vi "GeoData.vi"() -> ()   [LabVIEW 2017] (continued)
NY\tSuffolk County\tH1\n11752\t36103\tIslip terrace\tNY\tSuffolk County\tH1\n11767\t36103\tNesconset\tNY\tSuffolk County\tH1\n11780\t36103\tSaint james\tNY\tSuffolk County\tH1\n11776\t36103\tPort jefferson station\tNY\tSuffolk County\tH1\n11786\t36103\tShoreham\tNY\tSuffolk County\tH1\n11901\t36103\tRiverhead\tNY\tSuffolk County\tH1\n11942\t36103\tEast quogue\tNY\tSuffolk County\tH1\n11963\t36103\tSag harbor\tNY\tSuffolk County\tH1\n11940\t36103\tEast moriches\tNY\tSuffolk County\tH1\n11941\t36103\tEastport\tNY\tSuffolk County\tH1\n11962\t36103\tSagaponack\tNY\tSuffolk County\tH1\n11770\t36103\tOcean beach\tNY\tSuffolk County\tH1\n11965\t36103\tShelter island heights\tNY\tSuffolk County\tH1\n11947\t36103\tJamesport\tNY\tSuffolk County\tH1\n11706\t36103\tBay shore\tNY\tSuffolk County\tH1\n11720\t36103\tCentereach\tNY\tSuffolk County\tH1\n11718\t36103\tBrightwaters\tNY\tSuffolk County\tH1\n11763\t36103\tMedford\tNY\tSuffolk County\tH1\n11768\t36103\tNorthport\tNY\tSuffolk County\tH1\n11766\t36103\tMount sinai\tNY\tSuffolk County\tH1\n11779\t36103\tRonkonkoma\tNY\tSuffolk County\tH1\n11787\t36103\tSmithtown\tNY\tSuffolk County\tH1\n11937\t36103\tEast hampton\tNY\tSuffolk County\tH1\n11944\t36103\tGreenport\tNY\tSuffolk County\tH1\n11957\t36103\tOrient\tNY\tSuffolk County\tH1\n11954\t36103\tMontauk\tNY\tSuffolk County\tH1\n11960\t36103\tRemsenburg\tNY\tSuffolk County\tH1\n11969\t36103\tSouthampton\tNY\tSuffolk County\tH1\n11939\t36103\tEast marion\tNY\tSuffolk County\tH1\n11964\t36103\tShelter island\tNY\tSuffolk County\tH1\n12566\t36105\tPine bush\tNY\tSullivan County\tH1\n12742\t36105\tHarris\tNY\tSullivan County\tH1\n12732\t36105\tEldred\tNY\tSullivan County\tH1\n12745\t36105\tHortonville\tNY\tSullivan County\tH1\n12720\t36105\tBethel\tNY\tSullivan County\tH1\n12758\t36105\tLivingston manor\tNY\tSullivan County\tH1\n12458\t36105\tNapanoch\tNY\tSullivan County\tH1\n12762\t36105\tMongaup valley\tNY\tSullivan County\tH1\n12777\t36105\tForestburgh\tNY\tSullivan County\tH1\n12775\t36105\tRock hill\tNY\tSullivan County\tH1\n12763\t36105\tMountain dale\tNY\tSullivan County\tH1\n12743\t36105\tHighland lake\tNY\tSullivan County\tH1\n12767\t36105\tObernburg\tNY\tSullivan County\tH1\n12729\t36105\tCuddebackville\tNY\tSullivan County\tH1\n12748\t36105\tJeffersonville\tNY\tSullivan County\tH1\n12723\t36105\tCallicoon\tNY\tSullivan County\tH1\n12776\t36105\tRoscoe\tNY\tSullivan County\tH1\n12766\t36105\tNorth branch\tNY\tSullivan County\tH1\n12736\t36105\tFremont center\tNY\tSullivan County\tH1\n12722\t36105\tBurlingham\tNY\tSullivan County\tH1\n12721\t36105\tBloomingburg\tNY\tSullivan County\tH1\n12725\t36105\tClaryville\tNY\tSullivan County\tH1\n12726\t36105\tCochecton\tNY\tSullivan County\tH1\n12791\t36105\tYoungsville\tNY\tSullivan County\tH1\n12733\t36105\tFallsburg\tNY\tSullivan County\tH1\n12750\t36105\tKenoza lake\tNY\tSullivan County\tH1\n12724\t36105\tCallicoon center\tNY\tSullivan County\tH1\n12781\t36105\tSummitville\tNY\tSullivan County\tH1\n10940\t36105\tMiddletown\tNY\tSullivan County\tH1\n12701\t36105\tMonticello\tNY\tSullivan County\tH1\n12754\t36105\tLiberty\tNY\tSullivan County\tH1\n12741\t36105\tHankins\tNY\tSullivan County\tH1\n12738\t36105\tGlen wild\tNY\tSullivan County\tH1\n12783\t36105\tSwan lake\tNY\tSullivan County\tH1\n12740\t36105\tGrahamsville\tNY\tSullivan County\tH1\n12759\t36105\tLoch sheldrake\tNY\tSullivan County\tH1\n12786\t36105\tWhite lake\tNY\tSullivan County\tH1\n12787\t36105\tWhite sulphur springs\tNY\tSullivan County\tH1\n12435\t36105\tGreenfield park\tNY\tSullivan County\tH1\n12737\t36105\tGlen spey\tNY\tSullivan County\tH1\n12790\t36105\tWurtsboro\tNY\tSullivan County\tH1\n12768\t36105\tParksville\tNY\tSullivan County\tH1\n12779\t36105\tSouth fallsburg\tNY\tSullivan County\tH1\n12789\t36105\tWoodridge\tNY\tSullivan County\tH1\n12751\t36105\tKiamesha lake\tNY\tSullivan County\tH1\n12752\t36105\tLake huntington\tNY\tSullivan County\tH1\n12749\t36105\tKauneonga lake\tNY\tSullivan County\tH1\n12769\t36105\tPhillipsport\tNY\tSullivan County\tH1\n12784\t36105\tThompsonville\tNY\tSullivan County\tH1\n10963\t36105\tOtisville\tNY\tSullivan County\tH1\n12764\t36105\tNarrowsburg\tNY\tSullivan County\tH1\n12760\t36105\tLong eddy\tNY\tSullivan County\tH1\n12780\t36105\tSparrow bush\tNY\tSullivan County\tH1\n12788\t36105\tWoodbourne\tNY\tSullivan County\tH1\n12734\t36105\tFerndale\tNY\tSullivan County\tH1\n12765\t36105\tNeversink\tNY\tSullivan County\tH1\n12770\t36105\tPond eddy\tNY\tSullivan County\tH1\n12747\t36105\tHurleyville\tNY\tSullivan County\tH1\n12719\t36105\tBarryville\tNY\tSullivan County\tH1\n12792\t36105\tYulan\tNY\tSullivan County\tH1\n12778\t36105\tSmallwood\tNY\tSullivan County\tH1\n13850\t36107\tVestal\tNY\tTioga County\tH1\n13835\t36107\tRichford\tNY\tTioga County\tH1\n13864\t36107\tWillseyville\tNY\tTioga County\tH1\n13840\t36107\tSmithboro\tNY\tTioga County\tH1\n13845\t36107\tTioga center\tNY\tTioga County\tH1\n13732\t36107\tApalachin\tNY\tTioga County\tH1\n14889\t36107\tVan etten\tNY\tTioga County\tH1\n14883\t36107\tSpencer\tNY\tTioga County\tH1\n13734\t36107\tBarton\tNY\tTioga County\tH1\n13736\t36107\tBerkshire\tNY\tTioga County\tH1\n13811\t36107\tNewark valley\tNY\tTioga County\tH1\n13827\t36107\tOwego\tNY\tTioga County\tH1\n14859\t36107\tLockwood\tNY\tTioga County\tH1\n13743\t36107\tCandor\tNY\tTioga County\tH1\n13760\t36107\tEndicott\tNY\tTioga County\tH1\n14817\t36107\tBrooktondale\tNY\tTioga County\tH1\n14892\t36107\tWaverly\tNY\tTioga County\tH1\n13812\t36107\tNichols\tNY\tTioga County\tH1\n13053\t36109\tDryden\tNY\tTompkins County\tH1\n13092\t36109\tLocke\tNY\tTompkins County\tH1\n13864\t36109\tWillseyville\tNY\tTompkins County\tH1\n14867\t36109\tNewfield\tNY\tTompkins County\tH1\n14853\t36109\tIthaca\tNY\tTompkins County\tH1\n14883\t36109\tSpencer\tNY\tTompkins County\tH1\n13736\t36109\tBerkshire\tNY\tTompkins County\tH1\n14882\t36109\tLansing\tNY\tTompkins County\tH1\n13045\t36109\tCortland\tNY\tTompkins County\tH1\n13068\t36109\tFreeville\tNY\tTompkins County\tH1\n13073\t36109\tGroton\tNY\tTompkins County\tH1\n13062\t36109\tEtna\tNY\tTompkins County\tH1\n14854\t36109\tJacksonville\tNY\tTompkins County\tH1\n14817\t36109\tBrooktondale\tNY\tTompkins County\tH1\n14886\t36109\tTrumansburg\tNY\tTompkins County\tH1\n13081\t36109\tKing ferry\tNY\tTompkins County\tH1\n13102\t36109\tMc lean\tNY\tTompkins County\tH1\n14881\t36109\tSlaterville springs\tNY\tTompkins County\tH1\n14850\t36109\tIthaca\tNY\tTompkins County\tH1\n14851\t36109\tIthaca\tNY\tTompkins County\tH1\n14852\t36109\tIthaca\tNY\tTompkins County\tH1\n12455\t36111\tMargaretville\tNY\tUlster County\tH1\n12466\t36111\tPort ewen\tNY\tUlster County\tH1\n12443\t36111\tHurley\tNY\tUlster County\tH1\n12404\t36111\tAccord\tNY\tUlster County\tH1\n12494\t36111\tWest shokan\tNY\tUlster County\tH1\n12515\t36111\tClintondale\tNY\tUlster County\tH1\n12566\t36111\tPine bush\tNY\tUlster County\tH1\n13731\t36111\tAndes\tNY\tUlster County\tH1\n12409\t36111\tBearsville\tNY\tUlster County\tH1\n12589\t36111\tWallkill\tNY\tUlster County\tH1\n12406\t36111\tArkville\tNY\tUlster County\tH1\n12419\t36111\tCottekill\tNY\tUlster County\tH1\n12448\t36111\tLake hill\tNY\tUlster County\tH1\n12457\t36111\tMount tremper\tNY\tUlster County\tH1\n12588\t36111\tWalker valley\tNY\tUlster County\tH1\n12446\t36111\tKerhonkson\tNY\tUlster County\tH1\n12464\t36111\tPhoenicia\tNY\tUlster County\tH1\n12461\t36111\tOlivebridge\tNY\tUlster County\tH1\n12525\t36111\tGardiner\tNY\tUlster County\tH1\n12561\t36111\tNew paltz\tNY\tUlster County\tH1\n12586\t36111\tWalden\tNY\tUlster County\tH1\n12758\t36111\tLivingston manor\tNY\tUlster County\tH1\n12458\t36111\tNapanoch\tNY\tUlster County\tH1\n12471\t36111\tRifton\tNY\tUlster County\tH1\n12410\t36111\tBig indian\tNY\tUlster County\tH1\n12475\t36111\tRuby\tNY\tUlster County\tH1\n12417\t36111\tConnelly\tNY\tUlster County\tH1\n12428\t36111\tEllenville\tNY\tUlster County\tH1\n12472\t36111\tRosendale\tNY\tUlster County\tH1\n12481\t36111\tShokan\tNY\tUlster County\tH1\n12763\t36111\tMountain dale\tNY\tUlster County\tH1\n12441\t36111\tHighmount\tNY\tUlster County\tH1\n12548\t36111\tModena\tNY\tUlster County\tH1\n12490\t36111\tWest camp\tNY\tUlster County\tH1\n12486\t36111\tTillson\tNY\tUlster County\tH1\n12477\t36111\tSaugerties\tNY\tUlster County\tH1\n12414\t36111\tCatskill\tNY\tUlster County\tH1\n12402\t36111\tKingston\tNY\tUlster County\tH1\n12491\t36111\tWest hurley\tNY\tUlster County\tH1\n12542\t36111\tMarlboro\tNY\tUlster County\tH1\n12498\t36111\tWoodstock\tNY\tUlster County\tH1\n12487\t36111\tUlster park\tNY\tUlster County\tH1\n12725\t36111\tClaryville\tNY\tUlster County\tH1\n12433\t36111\tGlenford\tNY\tUlster County\tH1\n12480\t36111\tShandaken\tNY\tUlster County\tH1\n12456\t36111\tMount marion\tNY\tUlster County\tH1\n12429\t36111\tEsopus\tNY\tUlster County\tH1\n12401\t36111\tKingston\tNY\tUlster County\tH1\n12528\t36111\tHighland\tNY\tUlster County\tH1\n12465\t36111\tPine hill\tNY\tUlster County\tH1\n12740\t36111\tGrahamsville\tNY\tUlster County\tH1\n12453\t36111\tMalden on hudson\tNY\tUlster County\tH1\n12411\t36111\tBloomington\tNY\tUlster County\tH1\n12495\t36111\tWillow\tNY\tUlster County\tH1\n12435\t36111\tGreenfield park\tNY\tUlster County\tH1\n12432\t36111\tGlasco\tNY\tUlster County\tH1\n12483\t36111\tSpring glen\tNY\tUlster County\tH1\n12789\t36111\tWoodridge\tNY\tUlster County\tH1\n12489\t36111\tWawarsing\tNY\tUlster County\tH1\n12416\t36111\tChichester\tNY\tUlster County\tH1\n12568\t36111\tPlattekill\tNY\tUlster County\tH1\n12493\t36111\tWest park\tNY\tUlster County\tH1\n12420\t36111\tCragsmoor\tNY\tUlster County\tH1\n12463\t36111\tPalenville\tNY\tUlster County\tH1\n12440\t36111\tHigh falls\tNY\tUlster County\tH1\n12449\t36111\tLake katrine\tNY\tUlster County\tH1\n12484\t36111\tStone ridge\tNY\tUlster County\tH1\n12547\t36111\tMilton\tNY\tUlster County\tH1\n12412\t36111\tBoiceville\tNY\tUlster County\tH1\n12856\t36113\tNorth river\tNY\tWarren County\tH1\n12844\t36113\tKattskill bay\tNY\tWarren County\tH1\n12814\t36113\tBolton landing\tNY\tWarren County\tH1\n12885\t36113\tWarrensburg\tNY\tWarren County\tH1\n12817\t36113\tChestertown\tNY\tWarren County\tH1\n12878\t36113\tStony creek\tNY\tWarren County\tH1\n12810\t36113\tAthol\tNY\tWarren County\tH1\n12808\t36113\tAdirondack\tNY\tWarren County\tH1\n12835\t36113\tHadley\tNY\tWarren County\tH1\n12857\t36113\tOlmstedville\tNY\tWarren County\tH1\n12862\t36113\tRiparius\tNY\tWarren County\tH1\n12839\t36113\tHudson falls\tNY\tWarren County\tH1\n12824\t36113\tDiamond point\tNY\tWarren County\tH1\n12804\t36113\tQueensbury\tNY\tWarren County\tH1\n12815\t36113\tBrant lake\tNY\tWarren County\tH1\n12836\t36113\tHague\tNY\tWarren County\tH1\n12820\t36113\tCleverdale\tNY\tWarren County\tH1\n12870\t36113\tSchroon lake\tNY\tWarren County\tH1\n12886\t36113\tWevertown\tNY\tWarren County\tH1\n12845\t36113\tLake george\tNY\tWarren County\tH1\n12853\t36113\tNorth creek\tNY\tWarren County\tH1\n12843\t36113\tJohnsburg\tNY\tWarren County\tH1\n12860\t36113\tPottersville\tNY\tWarren County\tH1\n12874\t36113\tSilver bay\tNY\tWarren County\tH1\n12803\t36113\tSouth glens falls\tNY\tWarren County\tH1\n12801\t36113\tGlens falls\tNY\tWarren County\tH1\n12846\t36113\tLake luzerne\tNY\tWarren County\tH1\n12811\t36113\tBakers mills\tNY\tWarren County\tH1\n12828\t36115\tFort edward\tNY\tWashington County\tH1\n12883\t36115\tTiconderoga\tNY\tWashington County\tH1\n12841\t36115\tHuletts landing\tNY\tWashington County\tH1\n12844\t36115\tKattskill bay\tNY\tWashington County\tH1\n12185\t36115\tValley falls\tNY\tWashington County\tH1\n12849\t36115\tMiddle granville\tNY\tWashington County\tH1\n12028\t36115\tBuskirk\tNY\tWashington County\tH1\n12094\t36115\tJohnsonville\tNY\tWashington County\tH1\n12834\t36115\tGreenwich\tNY\tWashington County\tH1\n12838\t36115\tHartford\tNY\tWashington County\tH1\n12887\t36115\tWhitehall\tNY\tWashington County\tH1\n12837\t36115\tHampton\tNY\tWashington County\tH1\n12861\t36115\tPutnam station\tNY\tWashington County\tH1\n12823\t36115\tCossayuna\tNY\tWashington County\tH1\n12848\t36115\tMiddle falls\tNY\tWashington County\tH1\n12057\t36115\tEagle bridge\tNY\tWashington County\tH1\n12839\t36115\tHudson falls\tNY\tWashington County\tH1\n12804\t36115\tQueensbury\tNY\tWashington County\tH1\n12865\t36115\tSalem\tNY\tWashington County\tH1\n12873\t36115\tShushan\tNY\tWashington County\tH1\n12090\t36115\tHoosick falls\tNY\tWashington County\tH1\n12816\t36115\tCambridge\tNY\tWashington County\tH1\n12809\t36115\tArgyle\tNY\tWashington County\tH1\n12832\t36115\tGranville\tNY\tWashington County\tH1\n12821\t36115\tComstock\tNY\tWashington County\tH1\n12854\t36115\tNorth granville\tNY\tWashington County\tH1\n12827\t36115\tFort ann\tNY\tWashington County\tH1\n12154\t36115\tSchaghticoke\tNY\tWashington County\tH1\n12819\t36115\tClemons\tNY\tWashington County\tH1\n13143\t36117\tRed creek\tNY\tWayne County\tH1\n14433\t36117\tClyde\tNY\tWayne County\tH1\n14580\t36117\tWebster\tNY\tWayne County\tH1\n14563\t36117\tUnion hill\tNY\tWayne County\tH1\n14502\t36117\tMacedon\tNY\tWayne County\tH1\n14555\t36117\tSodus point\tNY\tWayne County\tH1\n14542\t36117\tRose\tNY\tWayne County\tH1\n14519\t36117\tOntario\tNY\tWayne County\tH1\n14413\t36117\tAlton\tNY\tWayne County\tH1\n13148\t36117\tSeneca falls\tNY\tWayne County\tH1\n14450\t36117\tFairport\tNY\tWayne County\tH1\n14589\t36117\tWilliamson\tNY\tWayne County\tH1\n13146\t36117\tSavannah\tNY\tWayne County\tH1\n14505\t36117\tMarion\tNY\tWayne County\tH1\n14513\t36117\tNewark\tNY\tWayne County\tH1\n13154\t36117\tSouth butler\tNY\tWayne County\tH1\n13156\t36117\tSterling\tNY\tWayne County\tH1\n14432\t36117\tClifton springs\tNY\tWayne County\tH1\n14489\t36117\tLyons\tNY\tWayne County\tH1\n14516\t36117\tNorth rose\tNY\tWayne County\tH1\n14522\t36117\tPalmyra\tNY\tWayne County\tH1\n14551\t36117\tSodus\tNY\tWayne County\tH1\n14538\t36117\tPultneyville\tNY\tWayne County\tH1\n13165\t36117\tWaterloo\tNY\tWayne County\tH1\n14532\t36117\tPhelps\tNY\tWayne County\tH1\n14590\t36117\tWolcott\tNY\tWayne County\tH1\n14568\t36117\tWalworth\tNY\tWayne County\tH1\n14520\t36117\tOntario center\tNY\tWayne County\tH1\n14449\t36117\tEast williamson\tNY\tWayne County\tH1\n10511\t36119\tBuchanan\tNY\tWestchester County\tH1\n10547\t36119\tMohegan lake\tNY\tWestchester County\tH1\n10580\t36119\tRye\tNY\tWestchester County\tH1\n10594\t36119\tThornwood\tNY\tWestchester County\tH1\n10601\t36119\tWhite plains\tNY\tWestchester County\tH1\n10704\t36119\tYonkers\tNY\tWestchester County\tH1\n10801\t36119\tNew rochelle\tNY\tWestchester County\tH1\n10466\t36119\tBronx\tNY\tWestchester County\tH1\n10510\t36119\tBriarcliff manor\tNY\tWestchester County\tH1\n10504\t36119\tArmonk\tNY\tWestchester County\tH1\n10550\t36119\tMount vernon\tNY\tWestchester County\tH1\n10528\t36119\tHarrison\tNY\tWestchester County\tH1\n10589\t36119\tSomers\tNY\tWestchester County\tH1\n10802\t36119\tNew rochelle\tNY\tWestchester County\tH1\n10535\t36119\tJefferson valley\tNY\tWestchester County\tH1\n10545\t36119\tMaryknoll\tNY\tWestchester County\tH1\n10507\t36119\tBedford hills\tNY\tWestchester County\tH1\n10509\t36119\tBrewster\tNY\tWestchester County\tH1\n10573\t36119\tPort chester\tNY\tWestchester County\tH1\n10605\t36119\tWhite plains\tNY\tWestchester County\tH1\n10706\t36119\tHastings on hudson\tNY\tWestchester County\tH1\n10710\t36119\tYonkers\tNY\tWestchester County\tH1\n10505\t36119\tBaldwin place\tNY\tWestchester County\tH1\n10520\t36119\tCroton on hudson\tNY\tWestchester County\tH1\n10514\t36119\tChappaqua\tNY\tWestchester County\tH1\n10502\t36119\tArdsley\tNY\tWestchester County\tH1\n10538\t36119\tLarchmont\tNY\tWestchester County\tH1\n10549\t36119\tMount kisco\tNY\tWestchester County\tH1\n10523\t36119\tElmsford\tNY\tWestchester County\tH1\n10536\t36119\tKatonah\tNY\tWestchester County\tH1\n10533\t36119\tIrvington\tNY\tWestchester County\tH1\n10570\t36119\tPleasantville\tNY\tWestchester County\tH1\n10578\t36119\tPurdys\tNY\tWestchester County\tH1\n10709\t36119\tEastchester\tNY\tWestchester County\tH1\n10560\t36119\tNorth salem\tNY\tWestchester County\tH1\n10526\t36119\tGoldens bridge\tNY\tWestchester County\tH1\n10587\t36119\tShenorock\tNY\tWestchester County\tH1\n10506\t36119\tBedford\tNY\tWestchester County\tH1\n10532\t36119\tHawthorne\tNY\tWestchester County\tH1\n10603\t36119\tWhite plains\tNY\tWestchester County\tH1\n10591\t36119\tTarrytown\tNY\tWestchester County\tH1\n10701\t36119\tYonkers\tNY\tWestchester County\tH1\n10607\t36119\tWhite plains\tNY\tWestchester County\tH1\n10597\t36119\tWaccabuc\tNY\tWestchester County\tH1\n10610\t36119\tWhite plains\tNY\tWestchester County\tH1\n10503\t36119\tArdsley on hudson\tNY\tWestchester County\tH1\n10470\t36119\tBronx\tNY\tWestchester County\tH1\n10475\t36119\tBronx\tNY\tWestchester County\tH1\n10543\t36119\tMamaroneck\tNY\tWestchester County\tH1\n10541\t36119\tMahopac\tNY\tWestchester County\tH1\n10527\t36119\tGranite springs\tNY\tWestchester County\tH1\n10583\t36119\tScarsdale\tNY\tWestchester County\tH1\n10553\t36119\tMount vernon\tNY\tWestchester County\tH1\n10805\t36119\tNew rochelle\tNY\tWestchester County\tH1\n10708\t36119\tBronxville\tNY\tWestchester County\tH1\n10707\t36119\tTuckahoe\tNY\tWestchester County\tH1\n10577\t36119\tPurchase\tNY\tWestchester County\tH1\n10548\t36119\tMontrose\tNY\tWestchester County\tH1\n10562\t36119\tOssining\tNY\tWestchester County\tH1\n10566\t36119\tPeekskill\tNY\tWestchester County\tH1\n10552\t36119\tMount vernon\tNY\tWestchester County\tH1\n10606\t36119\tWhite plains\tNY\tWestchester County\tH1\n10705\t36119\tYonkers\tNY\tWestchester County\tH1\n10703\t36119\tYonkers\tNY\tWestchester County\tH1\n10588\t36119\tShrub oak\tNY\tWestchester County\tH1\n10501\t36119\tAmawalk\tNY\tWestchester County\tH1\n10540\t36119\tLincolndale\tNY\tWestchester County\tH1\n10518\t36119\tCross river\tNY\tWestchester County\tH1\n10519\t36119\tCroton falls\tNY\tWestchester County\tH1\n10522\t36119\tDobbs ferry\tNY\tWestchester County\tH1\n10530\t36119\tHartsdale\tNY\tWestchester County\tH1\n10546\t36119\tMillwood\tNY\tWestchester County\tH1\n10567\t36119\tCortlandt manor\tNY\tWestchester County\tH1\n10576\t36119\tPound ridge\tNY\tWestchester County\tH1\n10595\t36119\tValhalla\tNY\tWestchester County\tH1\n10598\t36119\tYorktown heights\tNY\tWestchester County\tH1\n10590\t36119\tSouth salem\tNY\tWestchester County\tH1\n10604\t36119\tWest harrison\tNY\tWestchester County\tH1\n10803\t36119\tPelham\tNY\tWestchester County\tH1\n10702\t36119\tYonkers\tNY\tWestchester County\tH1\n10804\t36119\tNew rochelle\tNY\tWestchester County\tH1\n10537\t36119\tLake peekskill\tNY\tWestchester County\tH1\n10551\t36119\tMount vernon\tNY\tWestchester County\tH1\n10517\t36119\tCrompond\tNY\tWestchester County\tH1\n10602\t36119\tWhite plains\tNY\tWestchester County\tH1\n10596\t36119\tVerplanck\tNY\tWestchester County\tH1\n14052\t36121\tEast aurora\tNY\tWyoming County\tH1\n14525\t36121\tPavilion\tNY\tWyoming County\tH1\n14037\t36121\tCowlesville\tNY\tWyoming County\tH1\n14549\t36121\tSilver lake\tNY\tWyoming County\tH1\n14030\t36121\tChaffee\tNY\tWyoming County\tH1\n14083\t36121\tJava village\tNY\tWyoming County\tH1\n14569\t36121\tWarsaw\tNY\tWyoming County\tH1\n14039\t36121\tDale\tNY\tWyoming County\tH1\n14113\t36121\tNorth java\tNY\tWyoming County\tH1\n14082\t36121\tJava center\tNY\tWyoming County\tH1\n14004\t36121\tAlden\tNY\tWyoming County\tH1\n14066\t36121\tGainesville\tNY\tWyoming County\tH1\n14427\t36121\tCastile\tNY\tWyoming County\tH1\n14591\t36121\tWyoming\tNY\tWyoming County\tH1\n14040\t36121\tDarien center\tNY\tWyoming County\tH1\n14145\t36121\tStrykersville\tNY\tWyoming County\tH1\n14533\t36121\tPiffard\tNY\tWyoming County\tH1\n14024\t36121\tBliss\tNY\tWyoming County\tH1\n14054\t36121\tEast bethany\tNY\tWyoming County\tH1\n14481\t36121\tLeicester\tNY\tWyoming County\tH1\n14009\t36121\tArcade\tNY\tWyoming County\tH1\n14011\t36121\tAttica\tNY\tWyoming County\tH1\n14550\t36121\tSilver springs\tNY\tWyoming County\tH1\n14735\t36121\tFillmore\tNY\tWyoming County\tH1\n14130\t36121\tPike\tNY\tWyoming County\tH1\n14167\t36121\tVarysburg\tNY\tWyoming County\tH1\n14530\t36121\tPerry\tNY\tWyoming County\tH1\n14536\t36121\tPortageville\tNY\tWyoming County\tH1\n14857\t36123\tLakemont\tNY\tYates County\tH1\n14512\t36123\tNaples\tNY\tYates County\tH1\n14837\t36123\tDundee\tNY\tYates County\tH1\n14544\t36123\tRushville\tNY\tYates County\tH1\n14478\t36123\tKeuka park\tNY\tYates County\tH1\n14441\t36123\tDresden\tNY\tYates County\tH1\n14424\t36123\tCanandaigua\tNY\tYates County\tH1\n14873\t36123\tPrattsburgh\tNY\tYates County\tH1\n14842\t36123\tHimrod\tNY\tYates County\tH1\n14418\t36123\tBranchport\tNY\tYates County\tH1\n14561\t36123\tStanley\tNY\tYates County\tH1\n14507\t36123\tMiddlesex\tNY\tYates County\tH1\n14878\t36123\tRock stream\tNY\tYates County\tH1\n14527\t36123\tPenn yan\tNY\tYates County\tH1\n14456\t36123\tGeneva\tNY\tYates County\tH1\n14415\t36123\tBellona\tNY\tYates County\tH1\n27201\t37001\tAlamance\tNC\tAlamance County\tH1\n27349\t37001\tSnow camp\tNC\tAlamance County\tH1\n27202\t37001\tAltamahaw\tNC\tAlamance County\tH1\n27344\t37001\tSiler city\tNC\tAlamance County\tH1\n27217\t37001\tBurlington\tNC\tAlamance County\tH1\n27258\t37001\tHaw river\tNC\tAlamance County\tH1\n27302\t37001\tMebane\tNC\tAlamance County\tH1\n27340\t37001\tSaxapahaw\tNC\tAlamance County\tH1\n27244\t37001\tElon\tNC\tAlamance County\tH1\n27253\t37001\tGraham\tNC\tAlamance County\tH1\n27216\t37001\tBurlington\tNC\tAlamance County\tH1\n27298\t37001\tLiberty\tNC\tAlamance County\tH1\n27359\t37001\tSwepsonville\tNC\tAlamance County\tH1\n27215\t37001\tBurlington\tNC\tAlamance County\tH1\n27249\t37001\tGibsonville\tNC\tAlamance County\tH1\n28636\t37003\tHiddenite\tNC\tAlexander County\tH1\n28681\t37003\tTaylorsville\tNC\tAlexander County\tH1\n28630\t37003\tGranite falls\tNC\tAlexander County\tH1\n28654\t37003\tMoravian falls\tNC\tAlexander County\tH1\n28601\t37003\tHickory\tNC\tAlexander County\tH1\n28625\t37003\tStatesville\tNC\tAlexander County\tH1\n28678\t37003\tStony point\tNC\tAlexander County\tH1\n28689\t37003\tUnion grove\tNC\tAlexander County\tH1\n28644\t37005\tLaurel springs\tNC\tAlleghany County\tH1\n28663\t37005\tPiney creek\tNC\tAlleghany County\tH1\n28675\t37005\tSparta\tNC\tAlleghany County\tH1\n28668\t37005\tRoaring gap\tNC\tAlleghany County\tH1\n28627\t37005\tGlade valley\tNC\tAlleghany County\tH1\n28672\t37005\tScottville\tNC\tAlleghany County\tH1\n27017\t37005\tDobson\tNC\tAlleghany County\tH1\n28631\t37005\tGrassy creek\tNC\tAlleghany County\tH1\n28623\t37005\tEnnice\tNC\tAlleghany County\tH1\n28007\t37007\tAnsonville\tNC\tAnson County\tH1\n28135\t37007\tPolkton\tNC\tAnson County\tH1\n28119\t37007\tMorven\tNC\tAnson County\tH1\n28091\t37007\tLilesville\tNC\tAnson County\tH1\n28133\t37007\tPeachland\tNC\tAnson County\tH1\n28102\t37007\tMc farlan\tNC\tAnson County\tH1\n28103\t37007\tMarshville\tNC\tAnson County\tH1\n28170\t37007\tWadesboro\tNC\tAnson County\tH1\n28644\t37009\tLaurel springs\tNC\tAshe County\tH1\n28640\t37009\tJefferson\tNC\tAshe County\tH1\n28698\t37009\tZionville\tNC\tAshe County\tH1\n28629\t37009\tGlendale springs\tNC\tAshe County\tH1\n28643\t37009\tLansing\tNC\tAshe County\tH1\n28626\t37009\tFleetwood\tNC\tAshe County\tH1\n28618\t37009\tDeep gap\tNC\tAshe County\tH1\n28684\t37009\tTodd\tNC\tAshe County\tH1\n28693\t37009\tWarrensville\tNC\tAshe County\tH1\n28672\t37009\tScottville\tNC\tAshe County\tH1\n28694\t37009\tWest jefferson\tNC\tAshe County\tH1\n28617\t37009\tCrumpler\tNC\tAshe County\tH1\n28631\t37009\tGrassy creek\tNC\tAshe County\tH1\n28615\t37009\tCreston\tNC\tAshe County\tH1\n28622\t37011\tElk park\tNC\tAvery County\tH1\n28664\t37011\tPlumtree\tNC\tAvery County\tH1\n28653\t37011\tMontezuma\tNC\tAvery County\tH1\n28604\t37011\tBanner elk\tNC\tAvery County\tH1\n28777\t37011\tSpruce pine\tNC\tAvery County\tH1\n28646\t37011\tLinville\tNC\tAvery County\tH1\n28607\t37011\tBoone\tNC\tAvery County\tH1\n28605\t37011\tBlowing rock\tNC\tAvery County\tH1\n28662\t37011\tPineola\tNC\tAvery County\tH1\n28611\t37011\tCollettsville\tNC\tAvery County\tH1\n28652\t37011\tMinneapolis\tNC\tAvery County\tH1\n28616\t37011\tCrossnore\tNC\tAvery County\tH1\n28657\t37011\tNewland\tNC\tAvery County\tH1\n28679\t37011\tSugar grove\tNC\tAvery County\tH1\n28705\t37011\tBakersville\tNC\tAvery County\tH1\n27806\t37013\tAurora\tNC\tBeaufort County\tH1\n27860\t37013\tPantego\tNC\tBeaufort County\tH1\n27814\t37013\tBlounts creek\tNC\tBeaufort County\tH1\n27810\t37013\tBelhaven\tNC\tBeaufort County\tH1\n27962\t37013\tPlymouth\tNC\tBeaufort County\tH1\n28586\t37013\tVanceboro\tNC\tBeaufort County\tH1\n27821\t37013\tEdward\tNC\tBeaufort County\tH1\n27837\t37013\tGrimesland\tNC\tBeaufort County\tH1\n27889\t37013\tWashington\tNC\tBeaufort County\tH1\n27808\t37013\tBath\tNC\tBeaufort County\tH1\n27817\t37013\tChocowinity\tNC\tBeaufort County\tH1\n27834\t37013\tGreenville\tNC\tBeaufort County\tH1\n27871\t37013\tRobersonville\tNC\tBeaufort County\tH1\n27865\t37013\tPinetown\tNC\tBeaufort County\tH1\n27957\t37015\tMerry hill\tNC\tBertie County\tH1\n27983\t37015\tWindsor\tNC\tBertie County\tH1\n27805\t37015\tAulander\tNC\tBertie County\tH1\n27967\t37015\tPowellsville\tNC\tBertie County\tH1\n27924\t37015\tColerain\tNC\tBertie County\tH1\n27872\t37015\tRoxobel\tNC\tBertie County\tH1\n27869\t37015\tRich square\tNC\tBertie County\tH1\n27910\t37015\tAhoskie\tNC\tBertie County\tH1\n27849\t37015\tLewiston woodville\tNC\tBertie County\tH1\n27847\t37015\tKelford\tNC\tBertie County\tH1\n28320\t37017\tBladenboro\tNC\tBladen County\tH1\n28448\t37017\tKelly\tNC\tBladen County\tH1\n28444\t37017\tHarrells\tNC\tBladen County\tH1\n28306\t37017\tFayetteville\tNC\tBladen County\tH1\n28456\t37017\tRiegelwood\tNC\tBladen County\tH1\n28392\t37017\tTar heel\tNC\tBladen County\tH1\n28435\t37017\tCurrie\tNC\tBladen County\tH1\n28384\t37017\tSaint pauls\tNC\tBladen County\tH1\n28423\t37017\tBolton\tNC\tBladen County\tH1\n28337\t37017\tElizabethtown\tNC\tBladen County\tH1\n28382\t37017\tRoseboro\tNC\tBladen County\tH1\n28434\t37017\tCouncil\tNC\tBladen County\tH1\n28447\t37017\tIvanhoe\tNC\tBladen County\tH1\n28332\t37017\tDublin\tNC\tBladen County\tH1\n28312\t37017\tFayetteville\tNC\tBladen County\tH1\n28399\t37017\tWhite oak\tNC\tBladen County\tH1\n28433\t37017\tClarkton\tNC\tBladen County\tH1\n28438\t37017\tEvergreen\tNC\tBladen County\tH1\n28441\t37017\tGarland\tNC\tBladen County\tH1\n28422\t37019\tBolivia\tNC\tBrunswick County\tH1\n28467\t37019\tCalabash\tNC\tBrunswick County\tH1\n28470\t37019\tShallotte\tNC\tBrunswick County\tH1\n28452\t37019\tLongwood\tNC\tBrunswick County\tH1\n28436\t37019\tDelco\tNC\tBrunswick County\tH1\n28456\t37019\tRiegelwood\tNC\tBrunswick County\tH1\n28479\t37019\tWinnabow\tNC\tBrunswick County\tH1\n28401\t37019\tWilmington\tNC\tBrunswick County\tH1\n28451\t37019\tLeland\tNC\tBrunswick County\tH1\n28462\t37019\tSupply\tNC\tBrunswick County\tH1\n28469\t37019\tOcean isle beach\tNC\tBrunswick County\tH1\n28459\t37019\tShallotte\tNC\tBrunswick County\tH1\n28420\t37019\tAsh\tNC\tBrunswick County\tH1\n28461\t37019\tSouthport\tNC\tBrunswick County\tH1\n28465\t37019\tOak island\tNC\tBrunswick County\tH1\n28468\t37019\tSunset beach\tNC\tBrunswick County\tH1\n28701\t37021\tAlexander\tNC\tBuncombe County\tH1\n28715\t37021\tCandler\tNC\tBuncombe County\tH1\n28730\t37021\tFairview\tNC\tBuncombe County\tH1\n28814\t37021\tAsheville\tNC\tBuncombe County\tH1\n28655\t37021\tMorganton\tNC\tBuncombe County\tH1\n28714\t37021\tBurnsville\tNC\tBuncombe County\tH1\n28721\t37021\tClyde\tNC\tBuncombe County\tH1\n28804\t37021\tAsheville\tNC\tBuncombe County\tH1\n28757\t37021\tMontreat\tNC\tBuncombe County\tH1\n28770\t37021\tRidgecrest\tNC\tBuncombe County\tH1\n28709\t37021\tBarnardsville\tNC\tBuncombe County\tH1\n28732\t37021\tFletcher\tNC\tBuncombe County\tH1\n28762\t37021\tOld fort\tNC\tBuncombe County\tH1\n28806\t37021\tAsheville\tNC\tBuncombe County\tH1\n28776\t37021\tSkyland\tNC\tBuncombe County\tH1\n28805\t37021\tAsheville\tNC\tBuncombe County\tH1\n28803\t37021\tAsheville\tNC\tBuncombe County\tH1\n28802\t37021\tAsheville\tNC\tBuncombe County\tH1\n28704\t37021\tArden\tNC\tBuncombe County\tH1\n28778\t37021\tSwannanoa\tNC\tBuncombe County\tH1\n28787\t37021\tWeaverville\tNC\tBuncombe County\tH1\n28711\t37021\tBlack mountain\tNC\tBuncombe County\tH1\n28716\t37021\tCanton\tNC\tBuncombe County\tH1\n28801\t37021\tAsheville\tNC\tBuncombe County\tH1\n28816\t37021\tAsheville\tNC\tBuncombe County\tH1\n28813\t37021\tAsheville\tNC\tBuncombe County\tH1\n28815\t37021\tAsheville\tNC\tBuncombe County\tH1\n28810\t37021\tAsheville\tNC\tBuncombe County\tH1\n28753\t37021\tMarshall\tNC\tBuncombe County\tH1\n28748\t37021\tLeicester\tNC\tBuncombe County\tH1\n28754\t37021\tMars hill\tNC\tBuncombe County\tH1\n28791\t37021\tHendersonville\tNC\tBuncombe County\tH1\n28728\t37021\tEnka\tNC\tBuncombe County\tH1\n28759\t37021\tMills river\tNC\tBuncombe County\tH1\n28792\t37021\tHendersonville\tNC\tBuncombe County\tH1\n28602\t37023\tHickory\tNC\tBurke County\tH1\n28666\t37023\tIcard\tNC\tBurke County\tH1\n28619\t37023\tDrexel\tNC\tBurke County\tH1\n28645\t37023\tLenoir\tNC\tBurke County\tH1\n28655\t37023\tMorganton\tNC\tBurke County\tH1\n28761\t37023\tNebo\tNC\tBurke County\tH1\n28641\t37023\tJonas ridge\tNC\tBurke County\tH1\n28647\t37023\tLinville falls\tNC\tBurke County\tH1\n28671\t37023\tRutherford college\tNC\tBurke County\tH1\n28628\t37023\tGlen alpine\tNC\tBurke County\tH1\n28612\t37023\tConnelly springs\tNC\tBurke County\tH1\n28680\t37023\tMorganton\tNC\tBurke County\tH1\n28018\t37023\tBostic\tNC\tBurke County\tH1\n28601\t37023\tHickory\tNC\tBurke County\tH1\n28637\t37023\tHildebran\tNC\tBurke County\tH1\n28690\t37023\tValdese\tNC\tBurke County\tH1\n28168\t37023\tVale\tNC\tBurke County\tH1\n28657\t37023\tNewland\tNC\tBurke County\tH1\n28090\t37023\tLawndale\tNC\tBurke County\tH1\n28026\t37025\tConcord\tNC\tCabarrus County\tH1\n28269\t37025\tCharlotte\tNC\tCabarrus County\tH1\n28027\t37025\tConcord\tNC\tCabarrus County\tH1\n28075\t37025\tHarrisburg\tNC\tCabarrus County\tH1\n28213\t37025\tCharlotte\tNC\tCabarrus County\tH1\n28227\t37025\tCharlotte\tNC\tCabarrus County\tH1\n28083\t37025\tKannapolis\tNC\tCabarrus County\tH1\n28097\t37025\tLocust\tNC\tCabarrus County\tH1\n28071\t37025\tGold hill\tNC\tCabarrus County\tH1\n28107\t37025\tMidland\tNC\tCabarrus County\tH1\n28138\t37025\tRockwell\tNC\tCabarrus County\tH1\n28124\t37025\tMount pleasant\tNC\tCabarrus County\tH1\n28025\t37025\tConcord\tNC\tCabarrus County\tH1\n28036\t37025\tDavidson\tNC\tCabarrus County\tH1\n28081\t37025\tKannapolis\tNC\tCabarrus County\tH1\n28215\t37025\tCharlotte\tNC\tCabarrus County\tH1\n28082\t37025\tKannapolis\tNC\tCabarrus County\tH1\n28078\t37025\tHuntersville\tNC\tCabarrus County\tH1\n28262\t37025\tCharlotte\tNC\tCabarrus County\tH1\n28624\t37027\tFerguson\tNC\tCaldwell County\tH1\n28645\t37027\tLenoir\tNC\tCaldwell County\tH1\n28655\t37027\tMorganton\tNC\tCaldwell County\tH1\n28681\t37027\tTaylorsville\tNC\tCaldwell County\tH1\n28633\t37027\tLenoir\tNC\tCaldwell County\tH1\n28661\t37027\tPatterson\tNC\tCaldwell County\tH1\n28638\t37027\tHudson\tNC\tCaldwell County\tH1\n28630\t37027\tGranite falls\tNC\tCaldwell County\tH1\n28605\t37027\tBlowing rock\tNC\tCaldwell County\tH1\n28601\t37027\tHickory\tNC\tCaldwell County\tH1\n28611\t37027\tCollettsville\tNC\tCaldwell County\tH1\n28606\t37027\tBoomer\tNC\tCaldwell County\tH1\n28667\t37027\tRhodhiss\tNC\tCaldwell County\tH1\n27973\t37029\tShawboro\tNC\tCamden County\tH1\n27921\t37029\tCamden\tNC\tCamden County\tH1\n27974\t37029\tShiloh\tNC\tCamden County\tH1\n27909\t37029\tElizabeth city\tNC\tCamden County\tH1\n27976\t37029\tSouth mills\tNC\tCamden County\tH1\n28511\t37031\tAtlantic\tNC\tCarteret County\tH1\n28528\t37031\tGloucester\tNC\tCarteret County\tH1\n28570\t37031\tNewport\tNC\tCarteret County\tH1\n28582\t37031\tStella\tNC\tCarteret County\tH1\n28531\t37031\tHarkers island\tNC\tCarteret County\tH1\n28584\t37031\tSwansboro\tNC\tCarteret County\tH1\n28553\t37031\tMarshallberg\tNC\tCarteret County\tH1\n28516\t37031\tBeaufort\tNC\tCarteret County\tH1\n28555\t37031\tMaysville\tNC\tCarteret County\tH1\n28524\t37031\tDavis\tNC\tCarteret County\tH1\n28579\t37031\tSmyrna\tNC\tCarteret County\tH1\n28520\t37031\tCedar island\tNC\tCarteret County\tH1\n28575\t37031\tSalter path\tNC\tCarteret County\tH1\n28512\t37031\tAtlantic beach\tNC\tCarteret County\tH1\n28577\t37031\tSealevel\tNC\tCarteret County\tH1\n28557\t37031\tMorehead city\tNC\tCarteret County\tH1\n28594\t37031\tEmerald isle\tNC\tCarteret County\tH1\n28581\t37031\tStacy\tNC\tCarteret County\tH1\n28532\t37031\tHavelock\tNC\tCarteret County\tH1\n27315\t37033\tProvidence\tNC\tCaswell County\tH1\n27343\t37033\tSemora\tNC\tCaswell County\tH1\n27212\t37033\tBlanch\tNC\tCaswell County\tH1\n27326\t37033\tRuffin\tNC\tCaswell County\tH1\n27320\t37033\tReidsville\tNC\tCaswell County\tH1\n27217\t37033\tBurlington\tNC\tCaswell County\tH1\n27379\t37033\tYanceyville\tNC\tCaswell County\tH1\n27302\t37033\tMebane\tNC\tCaswell County\tH1\n27244\t37033\tElon\tNC\tCaswell County\tH1\n27314\t37033\tProspect hill\tNC\tCaswell County\tH1\n27305\t37033\tMilton\tNC\tCaswell County\tH1\n27249\t37033\tGibsonville\tNC\tCaswell County\tH1\n27291\t37033\tLeasburg\tNC\tCaswell County\tH1\n27311\t37033\tPelham\tNC\tCaswell County\tH1\n28602\t37035\tHickory\tNC\tCatawba County\tH1\n28092\t37035\tLincolnton\tNC\tCatawba County\tH1\n28658\t37035\tNewton\tNC\tCatawba County\tH1\n28609\t37035\tCatawba\tNC\tCatawba County\tH1\n28650\t37035\tMaiden\tNC\tCatawba County\tH1\n28612\t37035\tConnelly springs\tNC\tCatawba County\tH1\n28673\t37035\tSherrills ford\tNC\tCatawba County\tH1\n28037\t37035\tDenver\tNC\tCatawba County\tH1\n28682\t37035\tTerrell\tNC\tCatawba County\tH1\n28603\t37035\tHickory\tNC\tCatawba County\tH1\n28601\t37035\tHickory\tNC\tCatawba County\tH1\n28610\t37035\tClaremont\tNC\tCatawba County\tH1\n28168\t37035\tVale\tNC\tCatawba County\tH1\n28613\t37035\tConover\tNC\tCatawba County\tH1\n28090\t37035\tLawndale\tNC\tCatawba County\tH1\n27349\t37037\tSnow camp\tNC\tChatham County\tH1\n27207\t37037\tBear creek\tNC\tChatham County\tH1\n27330\t37037\tSanford\tNC\tChatham County\tH1\n27344\t37037\tSiler city\tNC\tChatham County\tH1\n27502\t37037\tApex\tNC\tChatham County\tH1\n27519\t37037\tCary\tNC\tChatham County\tH1\n27562\t37037\tNew hill\tNC\tChatham County\tH1\n27325\t37037\tRobbins\tNC\tChatham County\tH1\n27713\t37037\tDurham\tNC\tChatham County\tH1\n27355\t37037\tStaley\tNC\tChatham County\tH1\n27252\t37037\tGoldston\tNC\tChatham County\tH1\n27312\t37037\tPittsboro\tNC\tChatham County\tH1\n27516\t37037\tChapel hill\tNC\tChatham County\tH1\n27256\t37037\tGulf\tNC\tChatham County\tH1\n27213\t37037\tBonlee\tNC\tChatham County\tH1\n27332\t37037\tSanford\tNC\tChatham County\tH1\n27523\t37037\tApex\tNC\tChatham County\tH1\n27517\t37037\tChapel hill\tNC\tChatham County\tH1\n27208\t37037\tBennett\tNC\tChatham County\tH1\n27298\t37037\tLiberty\tNC\tChatham County\tH1\n27540\t37037\tHolly springs\tNC\tChatham County\tH1\n27559\t37037\tMoncure\tNC\tChatham County\tH1\n28901\t37039\tAndrews\tNC\tCherokee County\tH1\n28905\t37039\tMarble\tNC\tCherokee County\tH1\n28903\t37039\tCulberson\tNC\tCherokee County\tH1\n28906\t37039\tMurphy\tNC\tCherokee County\tH1\n28902\t37039\tBrasstown\tNC\tCherokee County\tH1\n27946\t37041\tHobbsville\tNC\tChowan County\tH1\n27919\t37041\tBelvidere\tNC\tChowan County\tH1\n27980\t37041\tTyner\tNC\tChowan County\tH1\n27932\t37041\tEdenton\tNC\tChowan County\tH1\n28734\t37043\tFranklin\tNC\tClay County\tH1\n28906\t37043\tMurphy\tNC\tClay County\tH1\n28904\t37043\tHayesville\tNC\tClay County\tH1\n28902\t37043\tBrasstown\tNC\tClay County\tH1\n28909\t37043\tWarne\tNC\tClay County\tH1\n28073\t37045\tGrover\tNC\tCleveland County\tH1\n28042\t37045\tFallston\tNC\tCleveland County\tH1\n28612\t37045\tConnelly springs\tNC\tCleveland County\tH1\n28150\t37045\tShelby\tNC\tCleveland County\tH1\n28151\t37045\tShelby\tNC\tCleveland County\tH1\n28136\t37045\tPolkville\tNC\tCleveland County\tH1\n28021\t37045\tCherryville\tNC\tCleveland County\tH1\n28020\t37045\tCasar\tNC\tCleveland County\tH1\n28168\t37045\tVale\tNC\tCleveland County\tH1\n28017\t37045\tBoiling springs\tNC\tCleveland County\tH1\n28169\t37045\tWaco\tNC\tCleveland County\tH1\n28089\t37045\tLattimore\tNC\tCleveland County\tH1\n28152\t37045\tShelby\tNC\tCleveland County\tH1\n28040\t37045\tEllenboro\tNC\tCleveland County\tH1\n28086\t37045\tKings mountain\tNC\tCleveland County\tH1\n28090\t37045\tLawndale\tNC\tCleveland County\tH1\n28114\t37045\tMooresboro\tNC\tCleveland County\tH1\n28038\t37045\tEarl\tNC\tCleveland County\tH1\n28320\t37047\tBladenboro\tNC\tColumbus County\tH1\n28463\t37047\tTabor city\tNC\tColumbus County\tH1\n28436\t37047\tDelco\tNC\tColumbus County\tH1\n28455\t37047\tNakina\tNC\tColumbus County\tH1\n28456\t37047\tRiegelwood\tNC\tColumbus County\tH1\n28424\t37047\tBrunswick\tNC\tColumbus County\tH1\n28423\t37047\tBolton\tNC\tColumbus County\tH1\n28430\t37047\tCerro gordo\tNC\tColumbus County\tH1\n28431\t37047\tChadbourn\tNC\tColumbus County\tH1\n28472\t37047\tWhiteville\tNC\tColumbus County\tH1\n28433\t37047\tClarkton\tNC\tColumbus County\tH1\n28438\t37047\tEvergreen\tNC\tColumbus County\tH1\n28442\t37047\tHallsboro\tNC\tColumbus County\tH1\n28432\t37047\tClarendon\tNC\tColumbus County\tH1\n28450\t37047\tLake waccamaw\tNC\tColumbus County\tH1\n28439\t37047\tFair bluff\tNC\tColumbus County\tH1\n28530\t37049\tGrifton\tNC\tCraven County\tH1\n28501\t37049\tKinston\tNC\tCraven County\tH1\n28527\t37049\tErnul\tNC\tCraven County\tH1\n28560\t37049\tNew bern\tNC\tCraven County\tH1\n28573\t37049\tPollocksville\tNC\tCraven County\tH1\n28586\t37049\tVanceboro\tNC\tCraven County\tH1\n28533\t37049\tCherry point\tNC\tCraven County\tH1\n28526\t37049\tDover\tNC\tCraven County\tH1\n28561\t37049\tNew bern\tNC\tCraven County\tH1\n28563\t37049\tNew bern\tNC\tCraven County\tH1\n28564\t37049\tNew bern\tNC\tCraven County\tH1\n28519\t37049\tBridgeton\tNC\tCraven County\tH1\n28523\t37049\tCove city\tNC\tCraven County\tH1\n28562\t37049\tNew bern\tNC\tCraven County\tH1\n28532\t37049\tHavelock\tNC\tCraven County\tH1\n28307\t37051\tFort bragg\tNC\tCumberland County\tH1\n28334\t37051\tDunn\tNC\tCumberland County\tH1\n28395\t37051\tWade\tNC\tCumberland County\tH1\n28302\t37051\tFayetteville\tNC\tCumberland County\tH1\n28342\t37051\tFalcon\tNC\tCumberland County\tH1\n28303\t37051\tFayetteville\tNC\tCumberland County\tH1\n28311\t37051\tFayetteville\tNC\tCumberland County\tH1\n28371\t37051\tParkton\tNC\tCumberland County\tH1\n28306\t37051\tFayetteville\tNC\tCumberland County\tH1\n28314\t37051\tFayetteville\tNC\tCumberland County\tH1\n28310\t37051\tFort bragg\tNC\tCumberland County\tH1\n28305\t37051\tFayetteville\tNC\tCumberland County\tH1\n28304\t37051\tFayetteville\tNC\tCumberland County\tH1\n28344\t37051\tGodwin\tNC\tCumberland County\tH1\n28384\t37051\tSaint pauls\tNC\tCumberland County\tH1\n28356\t37051\tLinden\tNC\tCumberland County\tH1\n28382\t37051\tRoseboro\tNC\tCumberland County\tH1\n28391\t37051\tStedman\tNC\tCumberland County\tH1\n28390\t37051\tSpring lake\tNC\tCumberland County\tH1\n28312\t37051\tFayetteville\tNC\tCumberland County\tH1\n28318\t37051\tAutryville\tNC\tCumberland County\tH1\n28348\t37051\tHope mills\tNC\tCumberland County\tH1\n28399\t37051\tWhite oak\tNC\tCumberland County\tH1\n28331\t37051\tCumberland\tNC\tCumberland County\tH1\n28301\t37051\tFayetteville\tNC\tCumberland County\tH1\n28441\t37051\tGarland\tNC\tCumberland County\tH1\n28309\t37051\tFayetteville\tNC\tCumberland County\tH1\n28308\t37051\tPope army airfield\tNC\tCumberland County\tH1\n27973\t37053\tShawboro\tNC\tCurrituck County\tH1\n27947\t37053\tJarvisburg\tNC\tCurrituck County\tH1\n27964\t37053\tPoint harbor\tNC\tCurrituck County\tH1\n27965\t37053\tPoplar branch\tNC\tCurrituck County\tH1\n27956\t37053\tMaple\tNC\tCurrituck County\tH1\n27923\t37053\tCoinjock\tNC\tCurrituck County\tH1\n27950\t37053\tKnotts island\tNC\tCurrituck County\tH1\n27929\t37053\t
